vi "Set Temp str (SubVI).vi"(9 "queue out":refnum<queue>, 10 "字符串":string) -> (0 "错误输出":errorcluster)   [LabVIEW 2019, in "Take Seq.lvlib"]
uses:
  Take Seq.lvlib
  config.ctl
  Instrument.ctl
  lib/QDInstrument.dll
  <vilib>/NI/Modbus Library/API/Master/Modbus Master.lvclass
  SubVI.lvlib
panel:
  # "(真是通道1，假是通道2)"
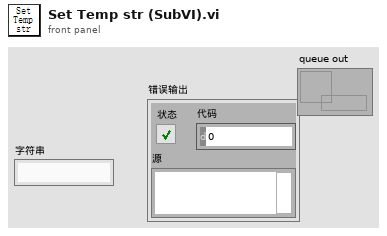
[diagram p1: front panel]
types:
  T1 = typedef "config.ctl" = cluster{"initialize":string, "6221":cluster{"6221 Resource":refnum<visa-resource-name>, "Delta status":bool}, "7001":cluster{"Ch":bool}, "SR830+6221":cluster{"source":u16, "阻抗":dbl, "量程入 4":i32, "量程入 3":i32, "量程入 2":i32, "量程入 1":i32, "电流":dbl, "SR830 2":bool, "SR830 3":bool, "SR830 4":bool, "SR830 1":bool, "VISA 1":refnum<visa-resource-name>, "VISA 2":refnum<visa-resource-name>, "VISA 3":refnum<visa-resource-name>, "VISA 4":refnum<visa-resource-name>, "量程":enum16{"量程每次测量会判定", "量程不变为设定值"}}, "2400":cluster{"2400":bool, "VISA":refnum<visa-resource-name>}, "ch":cluster{"ch str":string, "ch1":bool, "ch2":bool, "布尔":bool}, "error":bool, "数据文件路径":path, "log":cluster{"log路径":path, "log interval":dbl}, "Instrument":T2}
  T2 = typedef "Instrument.ctl" = cluster{"335 Resource":refnum<visa-resource-name>, "Input (0:A)":u16, "Instrument Type":i32, "quantum design":refnum<k24>, "Heater Output (1:1)":u16, "335state":refnum<vi>, "semaphore":T3, "TCP master instance":refnum<class "Modbus Master.lvclass">}
  T3 = typedef "Semaphore RefNum" = refnum<k1>
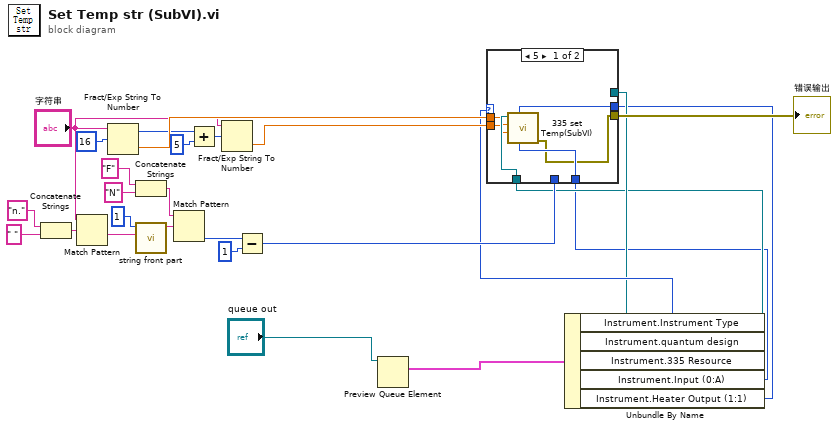
[diagram p0: block diagram]
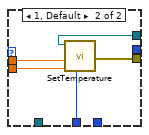
[diagram p2: hidden frame]
diagram:
  n1 = Concatenate Strings("n." ("正则表达式"), " " ("字符串")) -> (w26:string)
  n2 = Match Pattern(string="字符串", regular expression=w26) -> (after substring=w20:string)  [unwired: 1 in, 3 out]
  n3 = Fract/Exp String To Number(string="字符串", offset=16 ("偏移量")) -> (offset past number=w9:i32, number=w21:dbl)  [unwired: 2 in]
  n4 = Concatenate Strings("F" ("字符串"), "N" ("字符串")) -> (w16:string)
  n5 = call "string front part.vi"("字符串"=w20, "偏移量(0)"=1) -> ("result string"=w13:string)  [unwired: 9 in]
  n6 = Match Pattern(string=w16, regular expression=w13) -> (offset past match=w17:i32)  [unwired: 1 in, 3 out]
  n7 = Add(x=w9, y=5) -> (x+y=w10:i32)
  n8 = Fract/Exp String To Number(string="字符串", offset=w10) -> (number=w22:dbl)  [unwired: 2 in, 1 out]
  n9 = Subtract(x=w17, y=1) -> (x-y=w23:i32)
  n10 = Preview Queue Element(queue="queue out") -> (element=w6:T1)  [unwired: 2 in, 3 out]
  n11 = Unbundle By Name(w6) -> ("Instrument.Instrument Type"=w5:i32, "Instrument.quantum design"=w4:refnum<k24>, "Instrument.335 Resource"=w3:refnum<visa-resource-name>, "Instrument.Input (0:A)"=w2:u16, "Instrument.Heater Output (1:1)"=w1:u16)
  n12 = case shown="5" w5 {
    tunnel: [w29 w38] -> w27
    tunnel: w23 -> [_ w37]
    tunnel: w22 -> [w31 w36]
    tunnel: w21 -> [w30 w35]
    tunnel: w4 -> [_ w34]
    tunnel: w3 -> [w33 _]
    tunnel: w2 -> [w32 _]
    tunnel: w1 -> [w28 _]
    frame 5 {
      n13 = call "335 set Temp(SubVI).vi"("Input (0:A)"=w32, "Output (1:1)"=w28, "Rate"=w31, "Temperature"=w30, "VISA Refnum in"=w33) -> ("error out"=w29:errorcluster)  [unwired: 5 in, 1 out]
    }
    frame 1, Default {
      n14 = call "SetTemperature.vi"("Approach"=w37, "Rate"=w36, "Temperature"=w35, "Instrument Ref In"=w34) -> ("error out"=w38:errorcluster)  [unwired: 3 in, 2 out]
    }
  }
  "错误输出" <- w27
